vi "readU16FIFO.vi"(8 "error in (no error)":errorcluster, 9 "Timeout":i32, 10 "NumberOfElements":u32, 11 "ModbusRxDataFIFO in":refnum<class "ModbusRxDataFIFO.lvclass">) -> (0 "error out":errorcluster, 1 "ElementsRemaining":u32, 2 "Data":u16[](array[numeric]), 3 "ModbusRxDataFIFO out":refnum<class "ModbusRxDataFIFO.lvclass">)   [LabVIEW 2016, in "ModbusRxDataFIFO.lvclass"]
uses:
  ModbusRxDataFIFO.lvclass
  ModbusRxDataFIFO.lvclass/ModbusRxDataFIFO.ctl
  FPGA/FPGA.lvclass
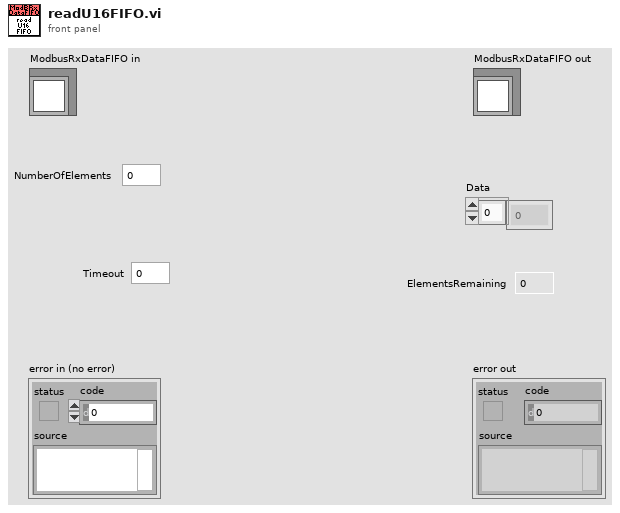
[diagram p1: front panel]
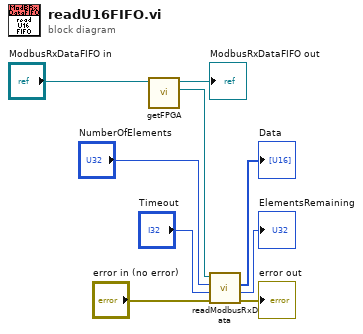
[diagram p0: block diagram]
diagram:
  n1 = call "getFPGA.vi"("ModbusRxDataFIFO in"="ModbusRxDataFIFO in") -> ("FPGA"=w8:refnum<class "FPGA.lvclass">, "ModbusRxDataFIFO out"=→"ModbusRxDataFIFO out":refnum<class "ModbusRxDataFIFO.lvclass">)  [unwired: 9 in]
  n2 = call "readModbusRxData.vi"("error in (no error)"="error in (no error)", "Timeout (ms)"="Timeout", "NumberOfElements"="NumberOfElements", "FPGA in"=w8) -> ("error out"=→"error out":errorcluster, "Elements Remaining"=→"ElementsRemaining":u32, "Data"=→"Data":u16[])  [unwired: 4 in, 1 out]
